vi "Get Number Photon Counting Divisions.vi"(8 "error in (no error)":errorcluster, 11 "noOfDivisions":u32) -> (0 "error out":errorcluster, 2 "function return":u32, 3 "noOfDivisions out":u32)   [LabVIEW 2014, in "atmcd32d.lvlib"]
doc: "unsigned int WINAPI GetNumberPhotonCountingDivisions(at_u32 * noOfDivisions);"
uses:
  atmcd32d.lvlib
  atmcd32d.dll
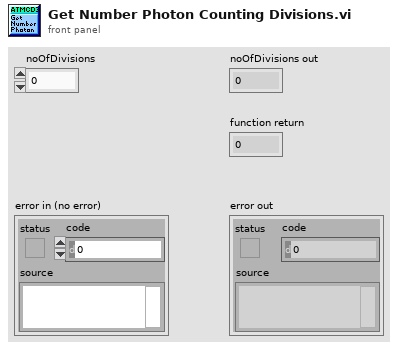
[diagram p1: front panel]
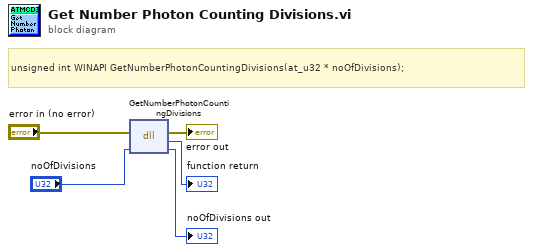
[diagram p0: block diagram]
diagram:
  # "unsigned int WINAPI GetNumberPhotonCountingDivisions(at_u32 * noOfDivisions);"
  n1 = dll-call lib="C:/Users/Bakir/Documents/Lambda2-Testing/lib/Andorlib/atmcd32d.*" fn="GetNumberPhotonCountingDivisions"(error in="error in (no error)", "noOfDivisions"="noOfDivisions") -> (error out=→"error out":errorcluster, →"function return":u32, "noOfDivisions"=→"noOfDivisions out":u32)  [unwired: 2 in, 1 out]
